vi "Delete Scale.vi"(8 "error in (no error)":errorcluster, 10 "index":i32, 11 "Scaling configuration in":refnum<class "Scaling configuration.lvclass">) -> (0 "error out":errorcluster, 3 "Scaling configuration out":refnum<class "Scaling configuration.lvclass">)   [LabVIEW 2013, in "Scaling configuration.lvclass"]
uses:
  Scaling configuration.lvclass
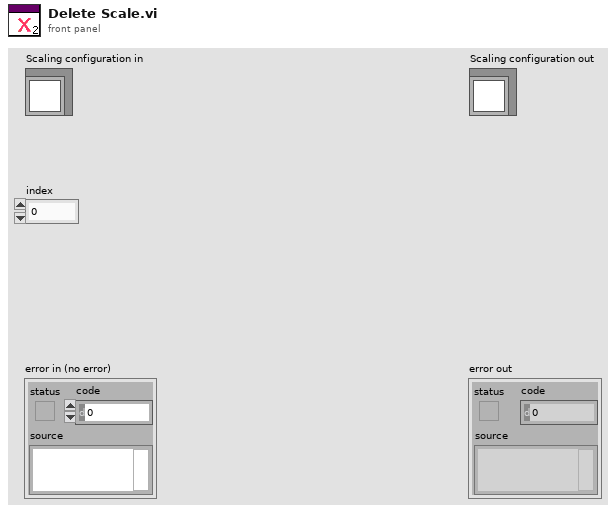
[diagram p1: front panel]
types:
  T1 = typedef "Scaling configuration.lvclass/scale data types.ctl" = enum16{"Double", "Single", "I64", "I32", "I16", "I8", "U64", "U32", "U16", "U8"}
  T2 = cluster{"mappings":cluster{"input channel":refnum<class "TBM channel.lvclass">, "output channel":refnum<class "TBM channel.lvclass">, "input data type":T1, "output data type":T1}[], "name":string}[]
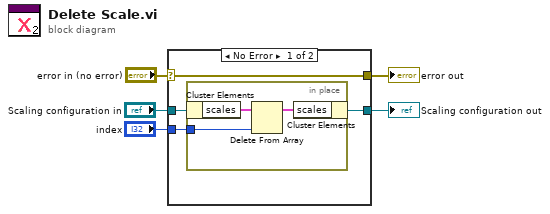
[diagram p0: block diagram]
diagram:
  n1 = case shown="No Error" "error in (no error)" {
    selector: "error in (no error)" -> [w6 w14]
    tunnel: [w6 w14] -> w4
    tunnel: [w7 w13] -> w2
    tunnel: "Scaling configuration in" -> [w9 w13]
    tunnel: "index" -> [w8 _]
    frame No Error {
      n2 = in-place {
        in-place-border: w8 -> [w11]
        n3 = in-place-cluster #1(w9) -> ("scales"=w12:T2)
        n4 = Delete From Array(array=w12, index=w11) -> (array with subset deleted=w10:T2)  [unwired: 1 in, 1 out]
        n5 = in-place-cluster #1("scales"=w10) -> (w7:refnum<class "Scaling configuration.lvclass">)
      }
    }
    frame Error {
    }
  }
  "error out" <- w4
  "Scaling configuration out" <- w2
